vi "User Event Print.vi"(7 "Options":T1, 8 "error in (no error)":errorcluster, 9 "add EOL? (T)":bool=TRUE, 11 "String to Print":string) -> (0 "error out":errorcluster, 3 "Print":refnum<user-event>)   [LabVIEW 2017]
uses:
  Print Options.ctl
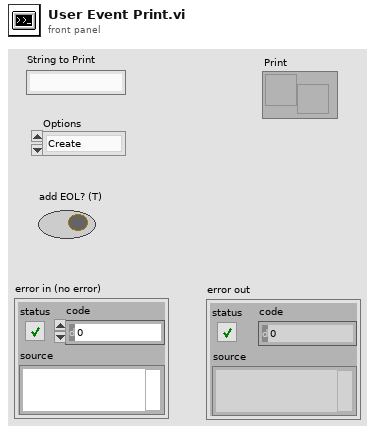
[diagram p1: front panel]
types:
  T1 = typedef "Print Options.ctl" = enum16{"Create", "Get Reference", "Print", "Print Header", "Close"}
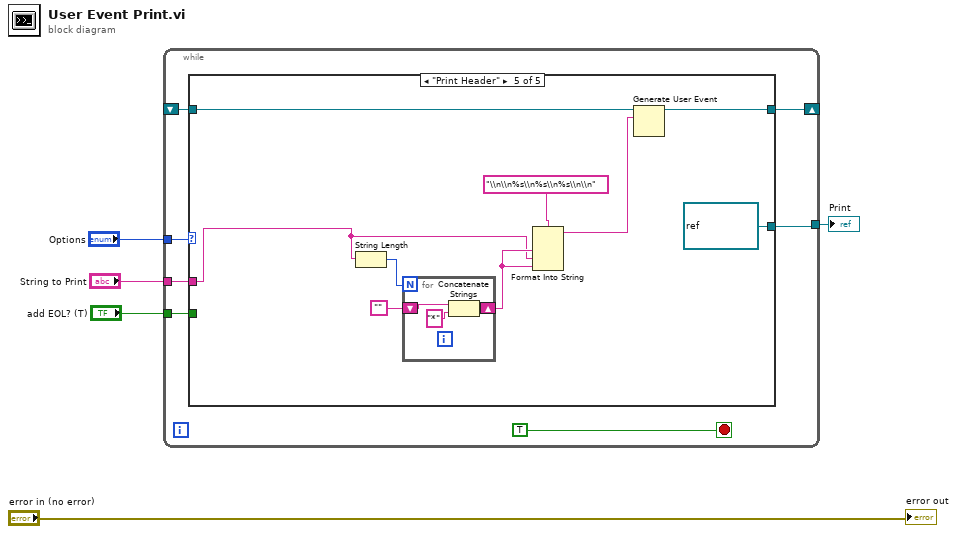
[diagram p0: block diagram]
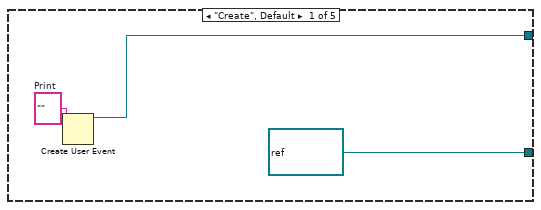
[diagram p2: hidden frame]
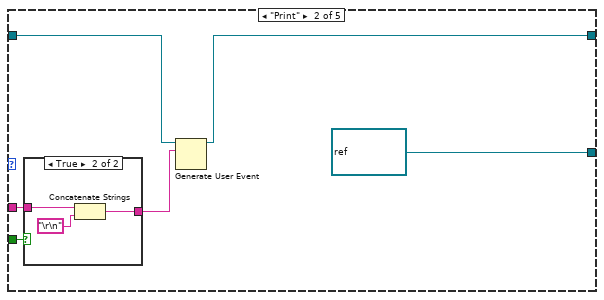
[diagram p3: hidden frame]
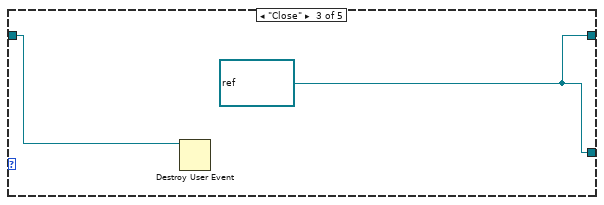
[diagram p5: hidden frame]
diagram:
  n1 = while {
    tunnel: "Options" -> [w11]
    tunnel: "String to Print" -> [w10]
    tunnel: "add EOL? (T)" -> [w9]
    shift-right: [w8] -> _
    shift-left: _ -> [w7]
    tunnel: [w6] -> w1
    stop <- TRUE stop-if-true
    n2 = case shown="\"Print Header\"" w11 {
      tunnel: w10 -> [_ w21 _ _ w29]
      tunnel: w9 -> [_ w19 _ _ _]
      tunnel: [w14 w17 w26 w28 w31] -> w8
      tunnel: w7 -> [_ w18 w27 w28 w37]
      tunnel: [refnum<user-event> refnum ("Print") refnum<user-event> refnum ("Print") w26 w28 refnum<user-event> refnum ("Print")] -> w6
      frame "Create", Default {
        w15 = ""  # Print
        n3 = Create User Event(user event datatype=w15) -> (user event=w14:refnum<user-event>)  [unwired: 1 in, 1 out]
      }
      frame "Print" {
        n4 = case shown="True" w19 {
          tunnel: w21 -> [w22 w25]
          tunnel: [w22 w24] -> w20
          frame False {
          }
          frame True {
            n5 = Concatenate Strings(w25, "\r\n") -> (w24:string)
          }
        }
        n6 = Generate User Event(user event=w18, event data cluster=w20) -> (user event out=w17:refnum<user-event>)  [unwired: 2 in, 1 out]
      }
      frame "Close" {
        w26 = refnum<user-event> refnum ("Print")
        n7 = Destroy User Event(user event=w27) -> ()  [unwired: 1 in, 1 out]
      }
      frame "Get Reference" {
      }
      frame "Print Header" {
        n8 = String Length(string=w29) -> (length=w35:i32)
        n9 = for {
          N: w35 -> [_]
          shift-right: [w38] -> w33
          shift-left: "" -> [w39]
          n10 = Concatenate Strings(w39, "*") -> (w38:string)
        }
        n11 = Format Into String(format string="\\n\\n%s\\n%s\\n%s\\n\\n", w33, w29, w33) -> (resulting string=w30:string)  [unwired: 2 in, 1 out]
        n12 = Generate User Event(user event=w37, event data cluster=w30) -> (user event out=w31:refnum<user-event>)  [unwired: 2 in, 1 out]
      }
    }
  }
  "Print" <- w1
  "error out" <- "error in (no error)"
